vi "Error_SetError.vi"(0 "QueueUpError?":bool=TRUE, 1 "status":bool, 2 "code (5000)":i32=5000, 3 "source":string, 5 "error in (no error)":errorcluster) -> (19 "error out":errorcluster)   [LabVIEW 2017]
doc: "You can use this VI to generate errors."
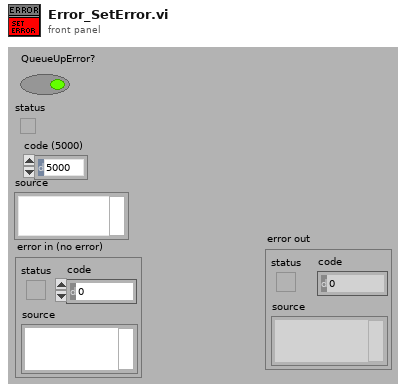
[diagram p1: front panel]
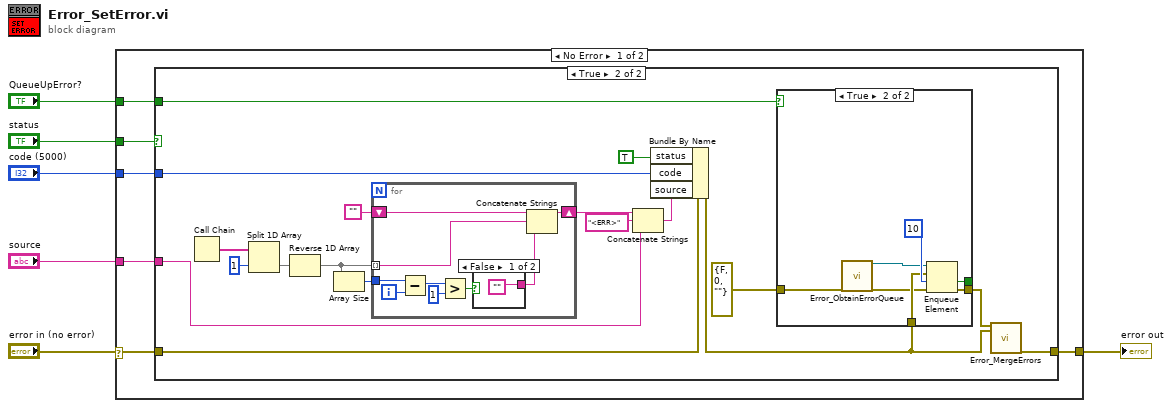
[diagram p0: block diagram]
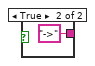
[diagram p4: hidden frame]
diagram:
  n1 = case shown="No Error" "error in (no error)" {
    selector: "error in (no error)" -> [w8 w51]
    tunnel: [w12 w51] -> w6
    tunnel: "status" -> [w11 _]
    tunnel: "code (5000)" -> [w10 _]
    tunnel: "source" -> [w9 _]
    tunnel: "QueueUpError?" -> [w7 _]
    frame No Error {
      n2 = case shown="True" w11 {
        tunnel: w8 -> [w13 w31]
        tunnel: [w13 w15] -> w12
        tunnel: w10 -> [_ w25]
        tunnel: w9 -> [_ w21]
        tunnel: w7 -> [_ w14]
        frame False {
        }
        frame True {
          n3 = Call Chain() -> (call chain=w29:string[])
          n4 = Split 1D Array(array=w29, index=1) -> (second subarray=w27:string[])  [unwired: 1 out]
          n5 = Reverse 1D Array(array=w27) -> (reversed array=w19:string[])
          n6 = Array Size(array=w19) -> (size(s)=w26:i32)
          n7 = for {
            shift-right: [w40] -> w23
            shift-left: "" -> [w43]
            tunnel: w19 -> [w41] mode=indexing
            tunnel: w26 -> [w48]
            i -> [w47]
            n8 = Subtract(x=w48, y=w47) -> (x-y=w46:i32)
            n9 = Greater?(x=w46, y=1) -> (0:w44:bool)
            n10 = case shown="False" w44 {
              tunnel: ["" "->"] -> w42
              frame False {
              }
              frame True {
              }
            }
            n11 = Concatenate Strings(w43, w41, w42) -> (w40:string)
          }
          n12 = Concatenate Strings(w23, "<ERR>" ("Substring"), w21) -> (w24:string)
          n13 = Bundle By Name(cluster=w31, "status"=TRUE ("Bundle Element"), "code"=w25, "source"=w24) -> (w17:errorcluster)
          n14 = case shown="True" w14 {
            tunnel: errorcluster {"status"=FALSE, "code"=0, "source"=""} ("error in (no error)") -> [w32 w36]
            tunnel: w17 -> [_ w38]
            tunnel: [w32 w37] -> w16
            tunnel: [_ w33] -> _
            frame False {
            }
            frame True {
              n15 = call "Error_ObtainErrorQueue.vi"("error in (no error)"=w36) -> ("ErrorQueue"=w34:refnum<queue>, "error out"=w35:errorcluster)  [unwired: 1 in, 16 out]
              n16 = Enqueue Element(queue=w34, element=w38, timeout in ms (-1)=10, error in (no error)=w35) -> (timed out?=w33:bool, error out=w37:errorcluster)  [unwired: 1 out]
            }
          }
          n17 = call "Error_MergeErrors.vi"("error in 1"=w16, "error in 2"=w17) -> ("error out"=w15:errorcluster)  [unwired: 1 in, 16 out]
        }
      }
    }
    frame Error {
    }
  }
  "error out" <- w6
